vi "TRG_SELECTOR - Type.vi"(8 "error in (no error)":errorcluster, 11 "TRG_SELECTOR":T1) -> (0 "error out":errorcluster, 3 "TRG_SELECTOR_VALUE":i32)   [LabVIEW 2018]
doc: "<b>Buffer policy settings can be only unsafe in xiAPI LabVIEW library</b>\nUNSAFE : User gets pointer to internally allocated circle buffer and data may be overwritten by device.\nSAFE : Data from device will be copied to user allocated buffer or xiApi allocated memory."
uses:
  TRG_SELECTOR.ctl
  C:/XIMEA/API/x64/xiApi.NETX64.dll
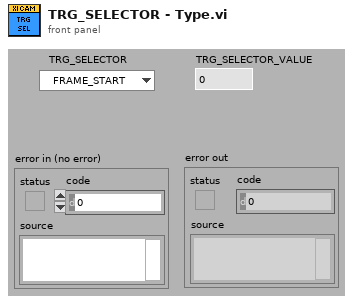
[diagram p1: front panel]
types:
  T1 = typedef "TRG_SELECTOR.ctl" = enum16{"FRAME_START", "EXPOSURE_ACTIVE", "FRAME_BURST_START", "FRAME_BURST_ACTIVE"}
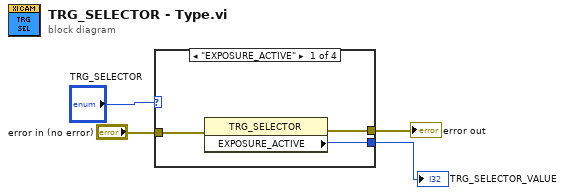
[diagram p0: block diagram]
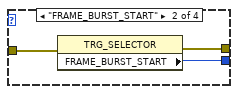
[diagram p2: hidden frame]
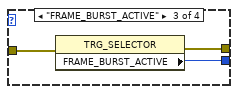
[diagram p3: hidden frame]
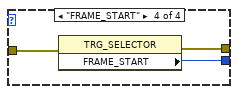
[diagram p4: hidden frame]
diagram:
  n1 = case shown="\"EXPOSURE_ACTIVE\"" "TRG_SELECTOR" {
    tunnel: "error in (no error)" -> [w7 w10 w13 w16]
    tunnel: [w6 w9 w12 w15] -> w3
    tunnel: [w5 w8 w11 w14] -> w2
    frame "EXPOSURE_ACTIVE" {
      n2 = property class="TRG_SELECTOR"(error in=w7) -> (error out=w6:errorcluster, "EXPOSURE_ACTIVE"=w5:i32)  [unwired: 1 in, 1 out]
    }
    frame "FRAME_BURST_START" {
      n3 = property class="TRG_SELECTOR"(error in=w10) -> (error out=w9:errorcluster, "FRAME_BURST_START"=w8:i32)  [unwired: 1 in, 1 out]
    }
    frame "FRAME_BURST_ACTIVE" {
      n4 = property class="TRG_SELECTOR"(error in=w13) -> (error out=w12:errorcluster, "FRAME_BURST_ACTIVE"=w11:i32)  [unwired: 1 in, 1 out]
    }
    frame "FRAME_START" {
      n5 = property class="TRG_SELECTOR"(error in=w16) -> (error out=w15:errorcluster, "FRAME_START"=w14:i32)  [unwired: 1 in, 1 out]
    }
  }
  "error out" <- w3
  "TRG_SELECTOR_VALUE" <- w2
